vi "Delta Time.vi"() -> (3 "dt (s)":dbl)   [LabVIEW 2014]
doc: "Returns time elapsed from previous call."
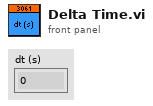
[diagram p1: front panel]
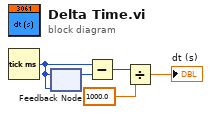
[diagram p0: block diagram]
diagram:
  n1 = Tick Count (ms)() -> (millisecond timer value=w4:u32)
  n2 = feedback-in #1(w4) -> ()
  n3 = feedback #1(w4) -> (w5:u32)
  n4 = Subtract(x=w4, y=w5) -> (x-y=w3:u32)
  n5 = Divide(x=w3, y=1000.0) -> (x/y=→"dt (s)":dbl)
